vi "Generate Grid Values.vi"(1 "Grid in":T1) -> (0 "Grid out":T1)   [LabVIEW 2023, in "NI_HFNetworkAnalysis.lvlib"]
doc: "Calculate grid values based on specified grid settings"
uses:
  NI_HFNetworkAnalysis.lvlib
  Controls/GridSettings.ctl
  Controls/ComplexConvention.ctl
  Controls/GridPatternType.ctl
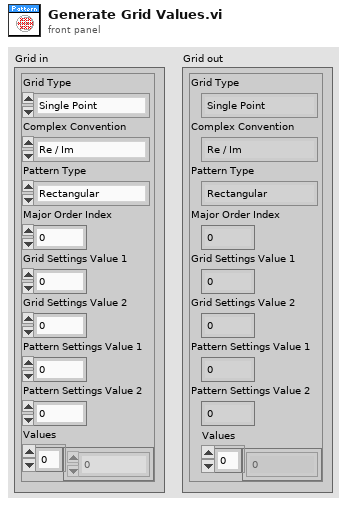
[diagram p1: front panel]
types:
  T1 = typedef "NI_HFNetworkAnalysis.lvlib/GridSettings.ctl" = cluster{"Grid Type":enum16{"Single Point", "Rectangle", "Circle", "Pie", "Custom"}, "Complex Convention":T2, "Pattern Type":T3, "Major Order Index":i32, "Grid Settings Value 1":cdb, "Grid Settings Value 2":cdb, "Pattern Settings Value 1":u32, "Pattern Settings Value 2":u32, "Values":cdb[]}
  T2 = typedef "NI_HFNetworkAnalysis.lvlib/ComplexConvention.ctl" = enum16{"Re / Im", "Amp / Pha"}
  T3 = typedef "NI_HFNetworkAnalysis.lvlib/GridPatternType.ctl" = enum16{"Rectangular", "Circular", "Undefined"}
  T4 = enum16{"Single Point", "Rectangle", "Circle", "Pie", "Custom"}
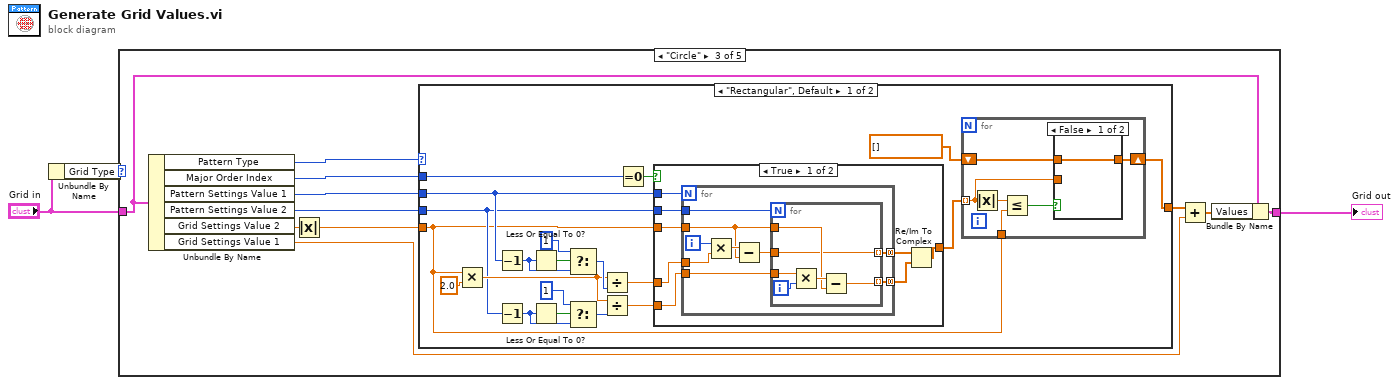
[diagram p0: block diagram]
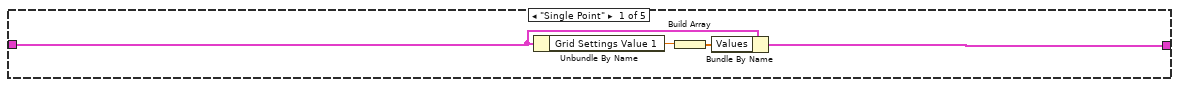
[diagram p2: hidden frame]
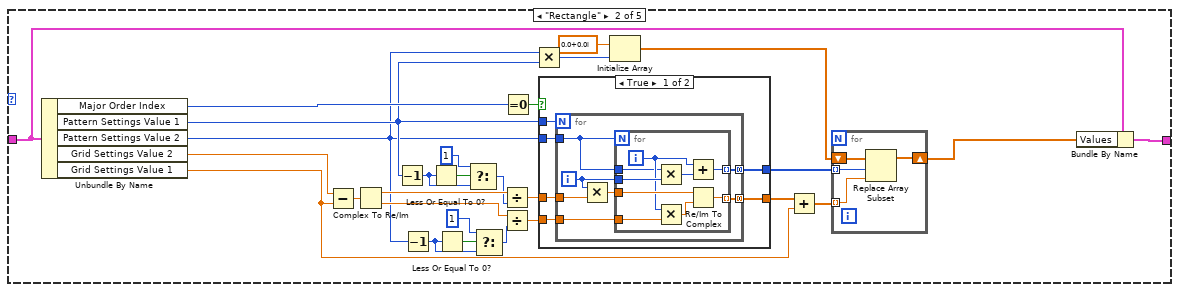
[diagram p3: hidden frame]
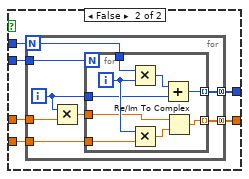
[diagram p4: hidden frame]
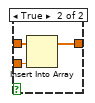
[diagram p5: hidden frame]
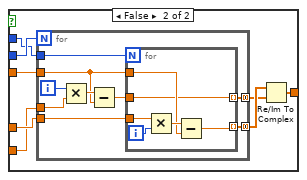
[diagram p6: hidden frame]
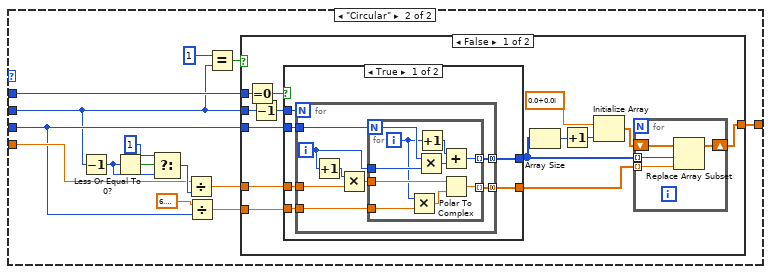
[diagram p7: hidden frame]
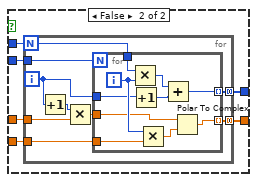
[diagram p8: hidden frame]
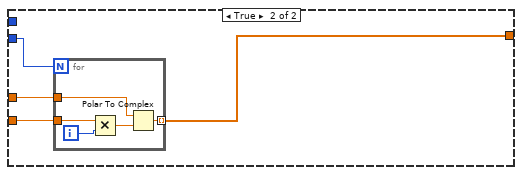
[diagram p9: hidden frame]
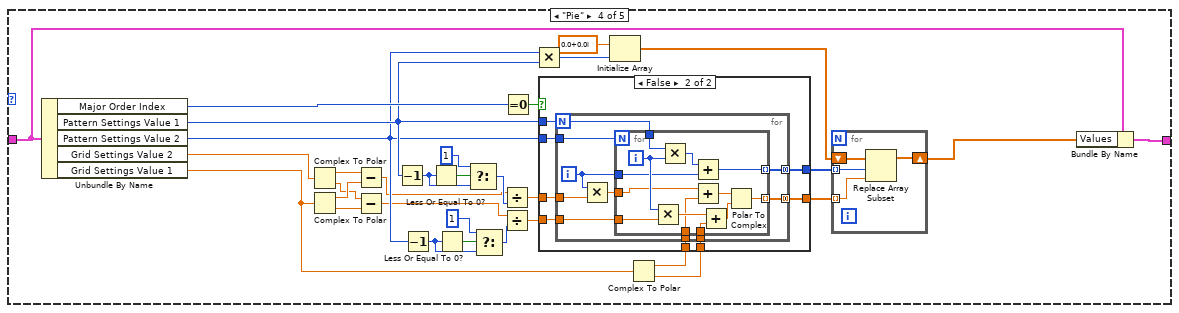
[diagram p10: hidden frame]
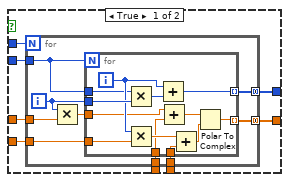
[diagram p11: hidden frame]
diagram:
  n1 = Unbundle By Name("Grid in") -> ("Grid Type"=w1:T4)
  n2 = case shown="\"Circle\"" w1 {
    tunnel: [w7 w27 w91 w286 w359] -> w3
    tunnel: "Grid in" -> [w4 w29 w92 w288 w359]
    frame "Single Point" {
      n3 = Unbundle By Name(w4) -> ("Grid Settings Value 1"=w5:cdb)
      n4 = Build Array(w5) -> (w6:cdb[])
      n5 = Bundle By Name(cluster=w4, "Values"=w6) -> (w7:T1)
    }
    frame "Rectangle" {
      n6 = Unbundle By Name(w29) -> ("Major Order Index"=w34:i32, "Pattern Settings Value 1"=w9:u32, "Pattern Settings Value 2"=w8:u32, "Grid Settings Value 2"=w23:cdb, "Grid Settings Value 1"=w22:cdb)
      n7 = Subtract(x=w23, y=w22) -> (x-y=w35:cdb)
      n8 = Complex To Re/Im(x + iy=w35) -> (x=w19:dbl, y=w18:dbl)
      n9 = Decrement(x=w9) -> (x-1=w12:u32)
      n10 = Decrement(x=w8) -> (x-1=w15:u32)
      n11 = Less Or Equal To 0?(x=w12) -> (x <= 0?=w13:bool)
      n12 = Less Or Equal To 0?(x=w15) -> (x <= 0?=w16:bool)
      n13 = Select(t=u32 1, s=w13, f=w12) -> (s? t:f=w11:u32)
      n14 = Select(t=u32 1, s=w16, f=w15) -> (s? t:f=w17:u32)
      n15 = Divide(x=w19, y=w11) -> (x/y=w21:dbl)
      n16 = Divide(x=w18, y=w17) -> (x/y=w20:dbl)
      n17 = Equal To 0?(x=w34) -> (x = 0?=w26:bool)
      n18 = Multiply(x=w8, y=w9) -> (x*y=w31:u32)
      n19 = case shown="True" w26 {
        tunnel: w20 -> [w36 w58]
        tunnel: w21 -> [w41 w59]
        tunnel: [w40 w63] -> w33
        tunnel: [w39 w62] -> w25
        tunnel: w9 -> [w37 w61]
        tunnel: w8 -> [w38 w60]
        frame True {
          n20 = for {
            N: w37 -> [_]
            tunnel: w38 -> [w48]
            tunnel: [w47] -> w40 mode=concatenating
            tunnel: w41 -> [w45]
            tunnel: w36 -> [w43]
            tunnel: [w42] -> w39 mode=concatenating
            i -> [w46]
            n21 = Multiply(x=w46, y=w45) -> (x*y=w44:dbl)
            n22 = for {
              N: w48 -> [_]
              tunnel: w48 -> [w50]
              tunnel: w46 -> [w57]
              tunnel: [w55] -> w47 mode=indexing
              tunnel: w44 -> [w53]
              tunnel: w43 -> [w54]
              tunnel: [w49] -> w42 mode=indexing
              i -> [w51]
              n23 = Multiply(x=w50, y=w57) -> (x*y=w56:u32)
              n24 = Multiply(x=w51, y=w54) -> (x*y=w52:dbl)
              n25 = Add(x=w51, y=w56) -> (x+y=w55:u32)
              n26 = Re/Im To Complex(1:w52, 2:w53) -> (0:w49:cdb)
            }
          }
        }
        frame False {
          n27 = for {
            N: w61 -> [w64]
            tunnel: w60 -> [w71]
            tunnel: [w70] -> w63 mode=concatenating
            tunnel: w59 -> [w68]
            tunnel: w58 -> [w66]
            tunnel: [w65] -> w62 mode=concatenating
            i -> [w69]
            n28 = Multiply(x=w69, y=w68) -> (x*y=w67:dbl)
            n29 = for {
              N: w71 -> [_]
              tunnel: w64 -> [w80]
              tunnel: w69 -> [w73]
              tunnel: [w78] -> w70 mode=indexing
              tunnel: w67 -> [w75]
              tunnel: w66 -> [w77]
              tunnel: [w72] -> w65 mode=indexing
              i -> [w76]
              n30 = Multiply(x=w80, y=w76) -> (x*y=w79:i32)
              n31 = Multiply(x=w76, y=w77) -> (x*y=w74:dbl)
              n32 = Add(x=w79, y=w73) -> (x+y=w78:i32)
              n33 = Re/Im To Complex(1:w74, 2:w75) -> (0:w72:cdb)
            }
          }
        }
      }
      n34 = Initialize Array(cdb 0.0+0.0i ("element"), w31) -> (w30:cdb[])
      n35 = Add(x=w25, y=w22) -> (x+y=w24:cdb[])
      n36 = for {
        tunnel: w33 -> [w82] mode=indexing
        tunnel: w24 -> [w83] mode=indexing
        shift-right: [w84] -> w28
        shift-left: w30 -> [w81]
        n37 = Replace Array Subset(array=w81, new element=w83, index=w82) -> (w84:cdb[])
      }
      n38 = Bundle By Name(cluster=w29, "Values"=w28) -> (w27:T1)
    }
    frame "Circle" {
      n39 = Unbundle By Name(w92) -> ("Pattern Type"=w88:T3, "Major Order Index"=w95:i32, "Pattern Settings Value 1"=w94:u32, "Pattern Settings Value 2"=w93:u32, "Grid Settings Value 2"=w90:cdb, "Grid Settings Value 1"=w85:cdb)
      n40 = Absolute Value(x=w90) -> (abs(x)=w89:dbl)
      n41 = case shown="\"Rectangular\", Default" w88 {
        tunnel: w95 -> [w115 w179]
        tunnel: w94 -> [w105 w176]
        tunnel: w93 -> [w104 w178]
        tunnel: [w98 w172] -> w87
        tunnel: w89 -> [w99 w182]
        frame "Rectangular", Default {
          n42 = Multiply(x=w99, y=2.0) -> (x*y=w106:dbl)
          n43 = Decrement(x=w105) -> (x-1=w109:u32)
          n44 = Decrement(x=w104) -> (x-1=w96:u32)
          n45 = Less Or Equal To 0?(x=w109) -> (x <= 0?=w110:bool)
          n46 = Less Or Equal To 0?(x=w96) -> (x <= 0?=w112:bool)
          n47 = Select(t=u32 1, s=w110, f=w109) -> (s? t:f=w108:u32)
          n48 = Select(t=u32 1, s=w112, f=w96) -> (s? t:f=w113:u32)
          n49 = Divide(x=w106, y=w108) -> (x/y=w103:dbl)
          n50 = Divide(x=w106, y=w113) -> (x/y=w102:dbl)
          n51 = Equal To 0?(x=w115) -> (x = 0?=w101:bool)
          n52 = case shown="True" w101 {
            tunnel: w105 -> [w133 w154]
            tunnel: w104 -> [w132 w155]
            tunnel: w103 -> [w131 w153]
            tunnel: w102 -> [w130 w152]
            tunnel: w99 -> [w129 w156]
            tunnel: [w126 w149] -> w100
            frame True {
              n53 = for {
                N: w133 -> [_]
                tunnel: w132 -> [w142]
                tunnel: w131 -> [w140]
                tunnel: w130 -> [w139]
                tunnel: w129 -> [w137]
                tunnel: [w136] -> w128 mode=concatenating
                tunnel: [w134] -> w127 mode=concatenating
                i -> [w141]
                n54 = Multiply(x=w141, y=w140) -> (x*y=w138:dbl)
                n55 = Subtract(x=w138, y=w137) -> (x-y=w135:dbl)
                n56 = for {
                  N: w142 -> [_]
                  tunnel: w139 -> [w147]
                  tunnel: w137 -> [w145]
                  tunnel: [w144] -> w136 mode=indexing
                  tunnel: w135 -> [w144]
                  tunnel: [w143] -> w134 mode=indexing
                  i -> [w148]
                  n57 = Multiply(x=w147, y=w148) -> (x*y=w146:dbl)
                  n58 = Subtract(x=w146, y=w145) -> (x-y=w143:dbl)
                }
              }
              n59 = Re/Im To Complex(1:w127, 2:w128) -> (0:w126:cdb[])
            }
            frame False {
              n60 = for {
                N: w155 -> [_]
                tunnel: w154 -> [w165]
                tunnel: w152 -> [w163]
                tunnel: w153 -> [w162]
                tunnel: w156 -> [w160]
                tunnel: [w159] -> w150 mode=concatenating
                tunnel: [w157] -> w151 mode=concatenating
                i -> [w164]
                n61 = Multiply(x=w164, y=w163) -> (x*y=w161:dbl)
                n62 = Subtract(x=w161, y=w160) -> (x-y=w158:dbl)
                n63 = for {
                  N: w165 -> [_]
                  tunnel: w162 -> [w170]
                  tunnel: w160 -> [w168]
                  tunnel: [w167] -> w159 mode=indexing
                  tunnel: w158 -> [w167]
                  tunnel: [w166] -> w157 mode=indexing
                  i -> [w171]
                  n64 = Multiply(x=w170, y=w171) -> (x*y=w169:dbl)
                  n65 = Subtract(x=w169, y=w168) -> (x-y=w166:dbl)
                }
              }
              n66 = Re/Im To Complex(1:w150, 2:w151) -> (0:w149:cdb[])
            }
          }
          n67 = for {
            tunnel: w100 -> [w116] mode=indexing
            tunnel: w99 -> [w120]
            shift-right: [w119] -> w98
            shift-left: cdb[] [] -> [w118]
            n68 = Absolute Value(x=w116) -> (abs(x)=w121:dbl)
            n69 = Less Or Equal?(x=w121, y=w120) -> (x <= y?=w117:bool)
            n70 = case shown="False" w117 {
              tunnel: [w122 w125] -> w119
              tunnel: w118 -> [w122 w124]
              tunnel: w116 -> [_ w123]
              frame False {
              }
              frame True {
                n71 = Insert Into Array(array=w124, new element=w123) -> (w125:cdb[])  [unwired: 1 in]
              }
            }
          }
        }
        frame "Circular" {
          n72 = Decrement(x=w176) -> (x-1=w184:u32)
          n73 = Less Or Equal To 0?(x=w184) -> (x <= 0?=w185:bool)
          n74 = Select(t=u32 1, s=w185, f=w184) -> (s? t:f=w183:u32)
          n75 = Divide(x=w182, y=w183) -> (x/y=w174:dbl)
          n76 = Divide(x=6.283185307179586, y=w178) -> (x/y=w173:dbl)
          n77 = Equal?(x=u32 1, y=w176) -> (x = y?=w177:bool)
          n78 = case shown="False" w177 {
            tunnel: w179 -> [w198 _]
            tunnel: w176 -> [w193 _]
            tunnel: w178 -> [w197 w256]
            tunnel: w174 -> [w196 w255]
            tunnel: w173 -> [w195 w254]
            tunnel: [w190 w253] -> w172
            frame False {
              n79 = Equal To 0?(x=w198) -> (x = 0?=w199:bool)
              n80 = Decrement(x=w193) -> (x-1=w194:u32)
              n81 = case shown="True" w199 {
                tunnel: w195 -> [w204 w228]
                tunnel: w196 -> [w209 w229]
                tunnel: [w208 w233] -> w186
                tunnel: [w207 w232] -> w189
                tunnel: w194 -> [w205 w231]
                tunnel: w197 -> [w206 w230]
                frame True {
                  n82 = for {
                    N: w205 -> [_]
                    tunnel: w206 -> [w217]
                    tunnel: [w216] -> w208 mode=concatenating
                    tunnel: w209 -> [w215]
                    tunnel: w204 -> [w213]
                    tunnel: [w212] -> w207 mode=concatenating
                    i -> [w210]
                    n83 = Increment(x=w210) -> (x+1=w211:i32)
                    n84 = Multiply(x=w211, y=w215) -> (x*y=w214:dbl)
                    n85 = for {
                      N: w217 -> [w220]
                      tunnel: w210 -> [w227]
                      tunnel: [w225] -> w216 mode=indexing
                      tunnel: w214 -> [w223]
                      tunnel: w213 -> [w224]
                      tunnel: [w221] -> w212 mode=indexing
                      i -> [w219]
                      n86 = Multiply(x=w219, y=w224) -> (x*y=w222:dbl)
                      n87 = Multiply(x=w220, y=w227) -> (x*y=w226:i32)
                      n88 = Increment(x=w219) -> (x+1=w218:i32)
                      n89 = Add(x=w218, y=w226) -> (x+y=w225:i32)
                      n90 = Polar To Complex(1:w222, 2:w223) -> (0:w221:cdb)
                    }
                  }
                }
                frame False {
                  n91 = for {
                    N: w231 -> [w236]
                    tunnel: w230 -> [w242]
                    tunnel: [w241] -> w233 mode=concatenating
                    tunnel: w229 -> [w240]
                    tunnel: w228 -> [w238]
                    tunnel: [w237] -> w232 mode=concatenating
                    i -> [w234]
                    n92 = Increment(x=w234) -> (x+1=w235:i32)
                    n93 = Multiply(x=w235, y=w240) -> (x*y=w239:dbl)
                    n94 = for {
                      N: w242 -> [_]
                      tunnel: w236 -> [w252]
                      tunnel: w234 -> [w244]
                      tunnel: [w250] -> w241 mode=indexing
                      tunnel: w239 -> [w247]
                      tunnel: w238 -> [w249]
                      tunnel: [w245] -> w237 mode=indexing
                      i -> [w248]
                      n95 = Multiply(x=w252, y=w248) -> (x*y=w251:i32)
                      n96 = Increment(x=w244) -> (x+1=w243:i32)
                      n97 = Multiply(x=w248, y=w249) -> (x*y=w246:dbl)
                      n98 = Add(x=w251, y=w243) -> (x+y=w250:i32)
                      n99 = Polar To Complex(1:w246, 2:w247) -> (0:w245:cdb)
                    }
                  }
                }
              }
              n100 = Array Size(array=w186) -> (size(s)=w188:i32)
              n101 = Increment(x=w188) -> (x+1=w187:i32)
              n102 = Initialize Array(cdb 0.0+0.0i ("element"), w187) -> (w191:cdb[])
              n103 = for {
                shift-right: [w200] -> w190
                shift-left: w191 -> [w203]
                tunnel: w186 -> [w202] mode=indexing
                tunnel: w189 -> [w201] mode=indexing
                n104 = Replace Array Subset(array=w203, new element=w201, index=w202) -> (w200:cdb[])
              }
            }
            frame True {
              n105 = for {
                N: w256 -> [_]
                tunnel: w255 -> [w259]
                tunnel: w254 -> [w261]
                tunnel: [w257] -> w253 mode=indexing
                i -> [w260]
                n106 = Multiply(x=w261, y=w260) -> (x*y=w258:dbl)
                n107 = Polar To Complex(1:w258, 2:w259) -> (0:w257:cdb)
              }
            }
          }
        }
      }
      n108 = Add(x=w87, y=w85) -> (x+y=w86:cdb[])
      n109 = Bundle By Name(cluster=w92, "Values"=w86) -> (w91:T1)
    }
    frame "Pie" {
      n110 = Unbundle By Name(w288) -> ("Major Order Index"=w293:i32, "Pattern Settings Value 1"=w273:u32, "Pattern Settings Value 2"=w272:u32, "Grid Settings Value 2"=w271:cdb, "Grid Settings Value 1"=w264:cdb)
      n111 = Complex To Polar(r * e^(i*theta)=w271) -> (r=w270:dbl, theta=w268:dbl)
      n112 = Complex To Polar(r * e^(i*theta)=w264) -> (r=w269:dbl, theta=w267:dbl)
      n113 = Subtract(x=w270, y=w269) -> (x-y=w266:dbl)
      n114 = Subtract(x=w268, y=w267) -> (x-y=w265:dbl)
      n115 = Decrement(x=w273) -> (x-1=w276:u32)
      n116 = Decrement(x=w272) -> (x-1=w279:u32)
      n117 = Less Or Equal To 0?(x=w276) -> (x <= 0?=w277:bool)
      n118 = Less Or Equal To 0?(x=w279) -> (x <= 0?=w280:bool)
      n119 = Select(t=u32 1, s=w277, f=w276) -> (s? t:f=w275:u32)
      n120 = Select(t=u32 1, s=w280, f=w279) -> (s? t:f=w281:u32)
      n121 = Divide(x=w266, y=w275) -> (x/y=w283:dbl)
      n122 = Divide(x=w265, y=w281) -> (x/y=w282:dbl)
      n123 = Equal To 0?(x=w293) -> (x = 0?=w285:bool)
      n124 = Multiply(x=w272, y=w273) -> (x*y=w290:u32)
      n125 = Initialize Array(cdb 0.0+0.0i ("element"), w290) -> (w289:cdb[])
      n126 = Complex To Polar(r * e^(i*theta)=w264) -> (r=w262:dbl, theta=w263:dbl)
      n127 = case shown="False" w285 {
        tunnel: w282 -> [w296 w326]
        tunnel: w283 -> [w301 w327]
        tunnel: [w300 w331] -> w292
        tunnel: [w299 w330] -> w284
        tunnel: w273 -> [w297 w329]
        tunnel: w272 -> [w298 w328]
        tunnel: w263 -> [w295 w325]
        tunnel: w262 -> [w294 w324]
        frame True {
          n128 = for {
            N: w297 -> [_]
            tunnel: w298 -> [w310]
            tunnel: [w309] -> w300 mode=concatenating
            tunnel: w301 -> [w307]
            tunnel: w296 -> [w305]
            tunnel: [w304] -> w299 mode=concatenating
            tunnel: w295 -> [w303]
            tunnel: w294 -> [w302]
            i -> [w308]
            n129 = Multiply(x=w308, y=w307) -> (x*y=w306:dbl)
            n130 = for {
              N: w310 -> [_]
              tunnel: w310 -> [w318]
              tunnel: w308 -> [w323]
              tunnel: [w321] -> w309 mode=indexing
              tunnel: w306 -> [w314]
              tunnel: w305 -> [w320]
              tunnel: [w317] -> w304 mode=indexing
              tunnel: w303 -> [w312]
              tunnel: w302 -> [w311]
              i -> [w319]
              n131 = Multiply(x=w318, y=w323) -> (x*y=w322:u32)
              n132 = Multiply(x=w319, y=w320) -> (x*y=w316:dbl)
              n133 = Add(x=w319, y=w322) -> (x+y=w321:u32)
              n134 = Add(x=w314, y=w311) -> (x+y=w313:dbl)
              n135 = Add(x=w316, y=w312) -> (x+y=w315:dbl)
              n136 = Polar To Complex(1:w315, 2:w313) -> (0:w317:cdb)
            }
          }
        }
        frame False {
          n137 = for {
            N: w329 -> [w334]
            tunnel: w328 -> [w341]
            tunnel: [w340] -> w331 mode=concatenating
            tunnel: w327 -> [w338]
            tunnel: w326 -> [w336]
            tunnel: [w335] -> w330 mode=concatenating
            tunnel: w325 -> [w333]
            tunnel: w324 -> [w332]
            i -> [w339]
            n138 = Multiply(x=w339, y=w338) -> (x*y=w337:dbl)
            n139 = for {
              N: w341 -> [_]
              tunnel: w334 -> [w354]
              tunnel: w339 -> [w349]
              tunnel: [w352] -> w340 mode=indexing
              tunnel: w337 -> [w343]
              tunnel: w336 -> [w351]
              tunnel: [w348] -> w335 mode=indexing
              tunnel: w333 -> [w345]
              tunnel: w332 -> [w342]
              i -> [w350]
              n140 = Multiply(x=w350, y=w351) -> (x*y=w347:dbl)
              n141 = Multiply(x=w354, y=w350) -> (x*y=w353:i32)
              n142 = Add(x=w353, y=w349) -> (x+y=w352:i32)
              n143 = Add(x=w343, y=w342) -> (x+y=w344:dbl)
              n144 = Add(x=w347, y=w345) -> (x+y=w346:dbl)
              n145 = Polar To Complex(1:w346, 2:w344) -> (0:w348:cdb)
            }
          }
        }
      }
      n146 = for {
        tunnel: w292 -> [w356] mode=indexing
        tunnel: w284 -> [w357] mode=indexing
        shift-right: [w358] -> w287
        shift-left: w289 -> [w355]
        n147 = Replace Array Subset(array=w355, new element=w357, index=w356) -> (w358:cdb[])
      }
      n148 = Bundle By Name(cluster=w288, "Values"=w287) -> (w286:T1)
    }
    frame "Custom", Default {
    }
  }
  "Grid out" <- w3
